vi "Rectangle.vi"(0 "Rectangle in":refnum<class "Rectangle.lvclass">, 1 "id":i32, 2 "x":i32, 3 "y":i32, 4 "width":i32, 5 "height":i32, 7 "error in (no error)":errorcluster) -> (20 "Rectangle out":refnum<class "Rectangle.lvclass">, 27 "error out":errorcluster)   [LabVIEW 2018, in "Rectangle.lvclass"]
uses:
  Rectangle.lvclass
  Rectangle.lvclass/Rectangle.ctl
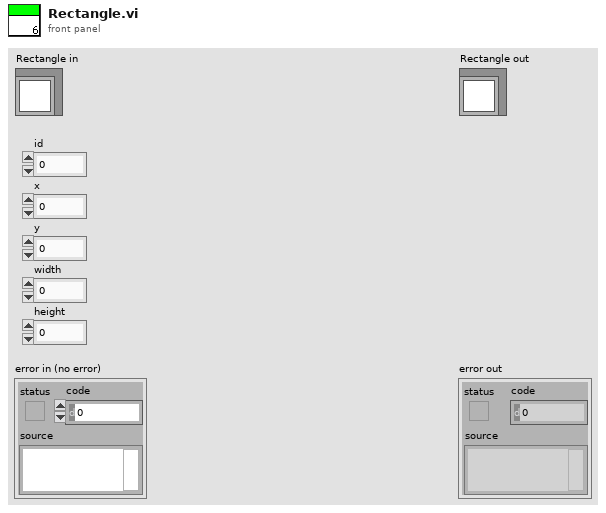
[diagram p1: front panel]
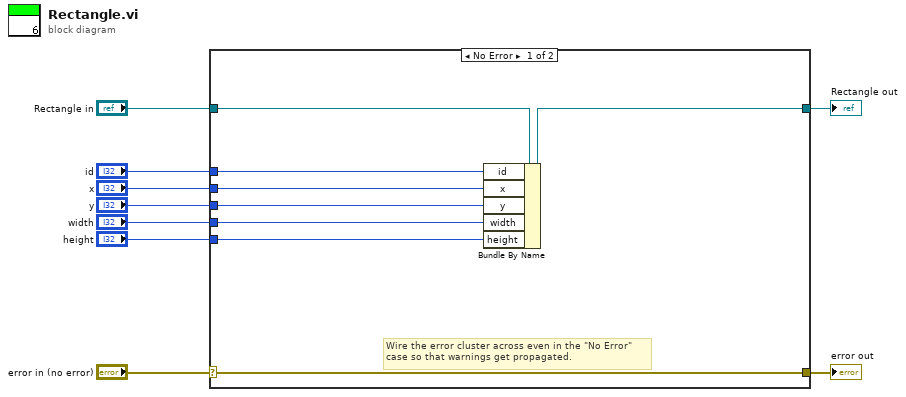
[diagram p0: block diagram]
diagram:
  n1 = case shown="No Error" "error in (no error)" {
    selector: "error in (no error)" -> [w16 w19]
    tunnel: [w16 w19] -> w8
    tunnel: [w15 w18] -> w6
    tunnel: "Rectangle in" -> [w17 w18]
    tunnel: "id" -> [w14 _]
    tunnel: "x" -> [w13 _]
    tunnel: "y" -> [w12 _]
    tunnel: "width" -> [w11 _]
    tunnel: "height" -> [w10 _]
    frame No Error {
      # "Wire the error cluster across even in the \"No Error\"\ncase so that warnings get propagated."
      n2 = Bundle By Name(cluster=w17, "id"=w14, "x"=w13, "y"=w12, "width"=w11, "height"=w10) -> (w15:refnum<class "Rectangle.lvclass">)
    }
    frame Error {
    }
  }
  "error out" <- w8
  "Rectangle out" <- w6
